vi "RT_Read_Analog_Input_FIFO_And_Stream.vi"(8 "error in (no error)":errorcluster, 10 "rt fifo":refnum<k33>, 11 "Network Stream endpoint":refnum<k21>) -> (0 "error out":errorcluster, 2 "Network Stream Timed Out":bool, 3 "endpoint out":refnum<k21>, 4 "Error FIFO":bool)   [LabVIEW 2020]
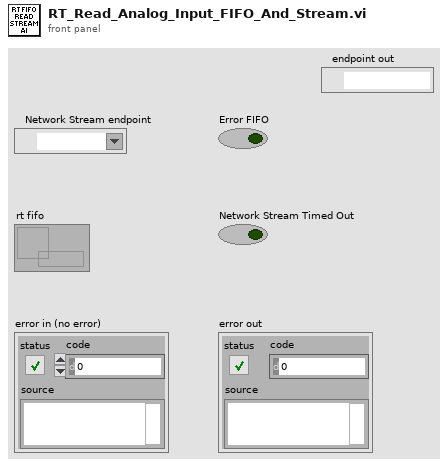
[diagram p1: front panel]
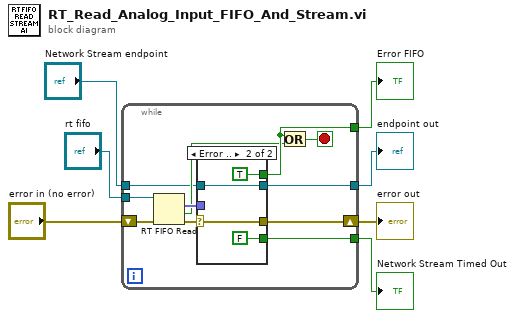
[diagram p0: block diagram]
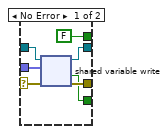
[diagram p2: hidden frame]
diagram:
  n1 = while {
    tunnel: "rt fifo" -> [w18]
    tunnel: [w17] -> w3
    tunnel: "Network Stream endpoint" -> [w11]
    shift-right: [w10] -> w6
    shift-left: "error in (no error)" -> [w12]
    tunnel: [w9] -> w7
    tunnel: [w8] -> w1
    stop <- w13 stop-if-true
    n2 = RT FIFO Read(0:w18, 3:w12) -> (9:w15:fxp<+/-,17,5>[], 10:w14:bool, 11:w16:errorcluster)  [unwired: 2 in, 2 out]
    n3 = case shown="Error .." w16 {
      selector: w16 -> [w22 w28]
      tunnel: w15 -> [w23 _]
      tunnel: [FALSE ("value") TRUE ("value")] -> w17
      tunnel: w11 -> [w24 w26]
      tunnel: [w21 w28] -> w10
      tunnel: [w20 FALSE] -> w9
      tunnel: [w19 w26] -> w8
      frame No Error {
        n4 = shared-variable-write(w24, w22, w23) -> (w19:refnum<k21>, w21:errorcluster, w20:bool)  [unwired: 1 in]
      }
      frame Error {
      }
    }
    n5 = Or(x=w17, y=w14) -> (x .or. y?=w13:bool)
  }
  "Network Stream Timed Out" <- w7
  "error out" <- w6
  "Error FIFO" <- w3
  "endpoint out" <- w1
